vi "Unreserve Device.vi"(8 "error in (no error)":errorcluster, 11 "SLSC Switch in":refnum<class "SLSC Switch.lvclass">) -> (0 "error out":errorcluster, 3 "SLSC Switch out":refnum<class "SLSC Switch.lvclass">)   [LabVIEW 2015, in "SLSC Switch.lvlib" / "SLSC Switch.lvclass"]
uses:
  SLSC Switch.lvclass
  <vilib>/National Instruments/SLSC Local or Remote Interface/SLSC Interface Class/SLSC Interface.lvclass
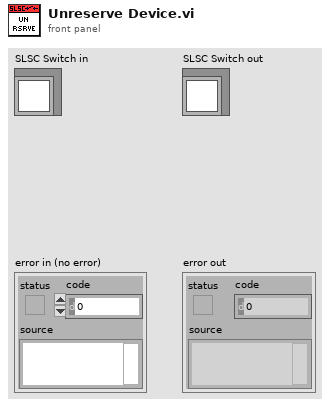
[diagram p1: front panel]
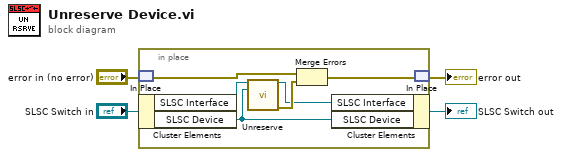
[diagram p0: block diagram]
diagram:
  n1 = in-place {
    n2 = in-place-match #1("error in (no error)") -> (w9:errorcluster)
    n3 = in-place-cluster #2("SLSC Switch in") -> ("SLSC Interface"=w6:refnum<class "SLSC Interface.lvclass">, "SLSC Device"=w10:refnum<k21>)
    n4 = call-dynamic "Unreserve.vi"("SLSC Interface in"=w6, "devices"=w10) -> ("SLSC Interface out"=w5:refnum<class "SLSC Interface.lvclass">, "error out"=w8:errorcluster)  [unwired: 12 in]
    n5 = Merge Errors(w9, w8) -> (w7:errorcluster)
    n6 = in-place-cluster #2("SLSC Interface"=w5, "SLSC Device"=w10) -> (→"SLSC Switch out":refnum<class "SLSC Switch.lvclass">)
    n7 = in-place-match #1(w7) -> (→"error out":errorcluster)
  }
